vi "Launcher.vi"(8 "error in (no error)":errorcluster, 10 "Levels to Spawn":i32=2, 11 "Actors/Level":i32=2) -> (0 "error out":errorcluster)   [LabVIEW 2020, in "Example Actor.lvlib" / "Example Actor.lvclass"]
doc: "Launcher launches the root-level actors as configured in the actor.\n\nCopyright (c) 2014, Moore Good Ideas, Inc.\n\nAll rights reserved.\n\nRedistribution and use in source and binary forms, with or without modification, are permitted provided that the following conditions are met:\n\n * Redistributions of source code must retain the above copyright notice, this list of conditions and the following disclaimer.\n * Redistributions in binary form must reproduce the above copyright notice, this list of conditions and the following disclaimer in the documentation and/or other materials provided with the distribution.\n * Neither the name of Moore Good Ideas, Inc. nor the names of its contributors may be used to endorse or promote products derived from this software without specific prior written permission.\n\nTHIS SOFTWARE IS PROVIDED BY THE COPYRIGHT HOLDERS AND CONTRIBUTORS \"AS IS\" AND ANY EXPRESS OR IMPLIED WARRANTIES, INCLUDING, BUT NOT LIMITED TO, THE IMPLIED WARRANTIES OF MERCHANTABILITY AND FITNESS FOR A PARTICULAR PURPOSE ARE DISCLAIMED. IN NO EVENT SHALL THE COPYRIGHT OWNER OR CONTRIBUTORS BE LIABLE FOR ANY DIRECT, INDIRECT, INCIDENTAL, SPECIAL, EXEMPLARY, OR CONSEQUENTIAL DAMAGES (INCLUDING, BUT NOT LIMITED TO, PROCUREMENT OF SUBSTITUTE GOODS OR SERVICES; LOSS OF USE, DATA, OR PROFITS; OR BUSINESS INTERRUPTION) HOWEVER CAUSED AND ON ANY THEORY OF LIABILITY, WHETHER IN CONTRACT, STRICT LIABILITY, OR TORT (INCLUDING NEGLIGENCE OR OTHERWISE) ARISING IN ANY WAY OUT OF THE USE OF THIS SOFTWARE, EVEN IF ADVISED OF THE POSSIBILITY OF SUCH DAMAGE."
uses:
  Example Actor.lvclass
  <vilib>/ActorFramework/Message Queue/Message Queue.lvclass/Message Queue.ctl
  C:/Program Files/National Instruments/LabVIEW 2020/vi.lib/ActorFramework/Actor/Actor.lvclass
  <vilib>/ActorFramework/Actor/Actor.lvclass
  <vilib>/ActorFramework/Message Queue/Message Queue.lvclass
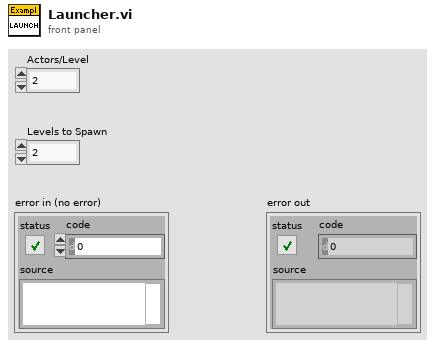
[diagram p1: front panel]
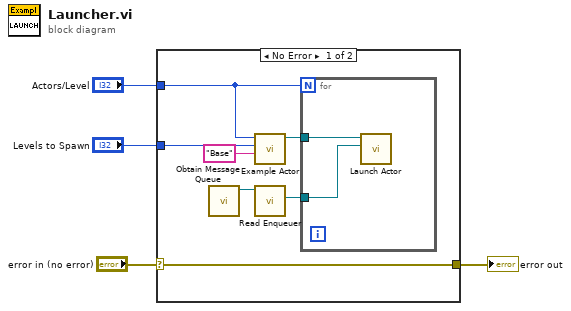
[diagram p0: block diagram]
diagram:
  n1 = case shown="No Error" "error in (no error)" {
    selector: "error in (no error)" -> [w5 w14]
    tunnel: "Levels to Spawn" -> [w8 _]
    tunnel: "Actors/Level" -> [w6 _]
    tunnel: [w5 w14] -> w2
    frame No Error {
      n2 = call <vilib>:"Obtain Message Queue.vi"() -> ("Message Queue"=w11:refnum<class "Message Queue.lvclass">)  [unwired: 10 in, 1 out]
      n3 = call "Example Actor.vi"("Parent ID"="Base", "Levels to Spawn"=w8, "Actors/Level"=w6) -> ("Example Actor out"=w9:refnum<class "Example Actor.lvclass">)  [unwired: 7 in, 1 out]
      n4 = call <vilib>:"Read Enqueuer.vi"("Message Queue"=w11) -> ("Message Enqueuer"=w10:refnum<class "Message Enqueuer.lvclass">)  [unwired: 10 in]
      n5 = for {
        N: w6 -> [_]
        tunnel: w9 -> [w13]
        tunnel: w10 -> [w12]
        n6 = call <vilib>:"Launch Actor.vi"("Actor-to-Caller Enqueuer"=w12, "Actor"=w13) -> ()  [unwired: 8 in, 2 out]
      }
    }
    frame Error {
    }
  }
  "error out" <- w2
